vi "Read Slewing Test Settings.vi"(8 "error in (no error)":errorcluster, 11 "Boot Loader in":refnum<class "Boot Loader.lvclass">) -> (0 "error out":errorcluster, 2 "Slewing Test Settings":T1 {"Settling Time (s)" format="%.4g"; "Hold Time (s)" format="%.4g"; "Ramp Time (s)" format="%.4g"; "Max Instance Force Error (N)" format="%.4g"; "Amplitude (N)" format="%.4g"; "Max Moment (NM)" format="%.4f"; "Max Force Error (N)" format="%.4f"}, 3 "Boot Loader out":refnum<class "Boot Loader.lvclass">)   [LabVIEW 2016, in "Boot Loader.lvclass"]
uses:
  Boot Loader.lvclass
  Typedefs/SlewingTestSettings.ctl
  Settings/Settings.lvclass
  Typedefs/FAMT Typedefs.lvlib
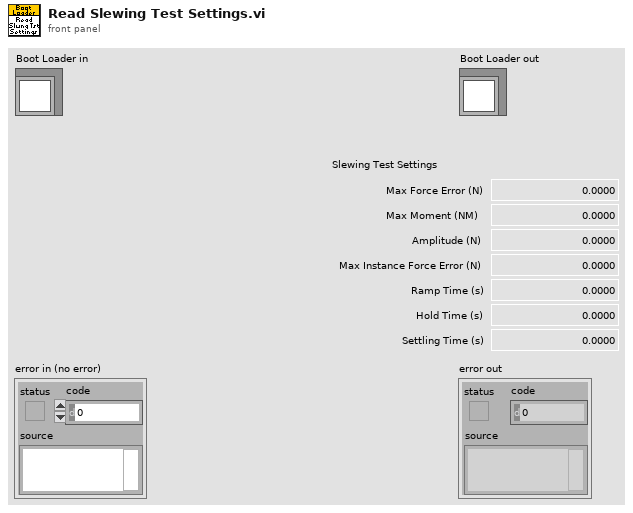
[diagram p1: front panel]
types:
  T1 = typedef "FAMT Typedefs.lvlib/SlewingTestSettings.ctl" = cluster{"Max Force Error (N)":dbl, "Max Moment (NM)":dbl, "Amplitude (N)":dbl, "Max Instance Force Error (N)":dbl, "Ramp Time (s)":dbl, "Hold Time (s)":dbl, "Settling Time (s)":dbl}
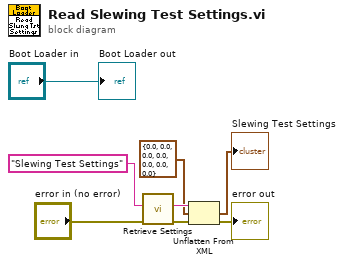
[diagram p0: block diagram]
diagram:
  n1 = call "Retrieve Settings.vi"("error in (no error)"="error in (no error)", "configName"="Slewing Test Settings") -> ("error out"=w4:errorcluster, "xmlConfig"=w7:string)  [unwired: 7 in, 1 out]
  n2 = Unflatten From XML(xml string=w7, type=T1 {"Max Force Error (N)"=0.0, "Max Moment (NM)"=0.0, "Amplitude (N)"=0.0, "Max Instance Force Error (N)"=0.0, "Ramp Time (s)"=0.0, "Hold Time (s)"=0.0, "Settling Time (s)"=0.0} ("Slewing Test Settings"), error in (no error)=w4) -> (value=→"Slewing Test Settings":T1, error out=→"error out":errorcluster)
  "Boot Loader out" <- "Boot Loader in"
